vi "DualDigitalOscilloscope .vi"() -> ()   [LabVIEW 2014]
panel:
  in  "Cluster":T1={"Number of Samples"=1000.0, "Sampling Frequency"=100000.0}
  out "Waveform Graph":dynamicdata(graph)=[{"t0"=timestamp(3496174688.203299 s since 1904-01-01), "dt"=9.999999999999972e-06, "Y"=array[1000 elements], "attributes"=variant("NI_ChannelName"=variant(string "Voltage"), "NI_UnitDescription"=variant(string "Volts"))}, {"t0"=timestamp(3496174688.203304 s since 1904-01-01), "dt"=9.999999999999972e-06, "Y"=array[1000 elements], "attributes"=variant("NI_ChannelName"=variant(string "Voltage_0"), "NI_UnitDescription"=variant(string "Volts"))}]
  out "error out":errorcluster
  in  "stop":bool
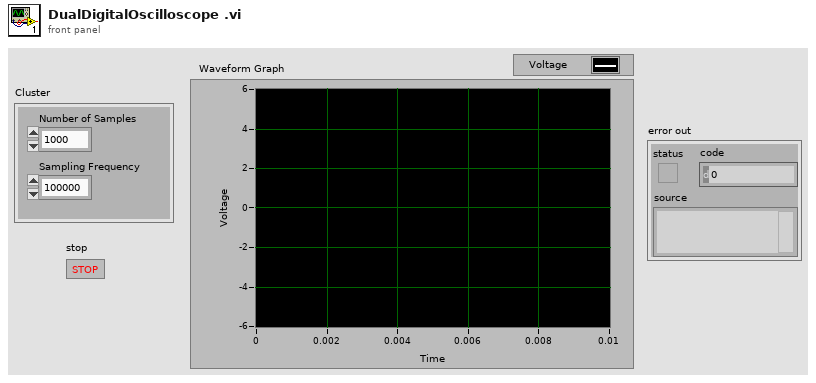
[diagram p1: front panel]
types:
  T1 = cluster{"Number of Samples":dbl, "Sampling Frequency":dbl}
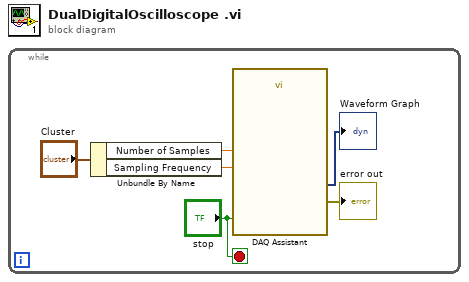
[diagram p0: block diagram]
diagram:
  n1 = while {
    stop <- "stop" stop-if-true
    n2 = Unbundle By Name("Cluster") -> ("Number of Samples"=w5:dbl, "Sampling Frequency"=w4:dbl)
    n3 = call "DAQ Assistant"("rate"=w4, "number of samples"=w5, "stop (T)"="stop") -> ("data"=→"Waveform Graph":dynamicdata, "error out"=→"error out":errorcluster)  [unwired: 14 in, 1 out]
  }
